vi "Target_long_compile.vi"() -> ()   [LabVIEW 2019]
uses:
  <vilib>/Platform/TimedLoop/XDataNode/timing_clust.ctl
  <vilib>/Platform/TimedLoop/XDataNode/nitl_modes.ctl
  <vilib>/Platform/TimedLoop/XDataNode/wakeup.ctl
  <vilib>/rvi/Emulation/niFpgaSctlEmulationGetInTimedLoop.vi
  <vilib>/rvi/Emulation/niFpgaEmulationReportErrorSimple.vi
  <vilib>/rvi/Emulation/niFpgaGetClockAttributes.vi
  <vilib>/rvi/Emulation/niFpgaCriticalErrorInLSC.vi
  <vilib>/rvi/DataTransferAndStorage/Container/Common/niFpgaContainerExecOnDevCompGetState.vi
  <vilib>/rvi/Emulation/niFpgaEmulationIsFPGAContextNoSignature.vi
  <vilib>/rvi/errors/niFpgaSetErrorForExecOnDevCompSimple.vi
  <vilib>/rvi/eio/common/nirviEmuReportErrorAndStop.vi
  <vilib>/rvi/DataTransferAndStorage/Container/Common/niFpgaContainerGetUniqueNameForEmu.vi
  <vilib>/rvi/FIFO/Fifo_Resource/nirvififoEmulationSetSize.vi
  <vilib>/rvi/FIFO/Fifo_Resource/nirviFifoEmulationQueueMgr.vi
  <instcachedir>/0/nirviFifoEmulationQueueMgr_E5CAEC123FF24DC58D834DCA3CDAA9B5.lvgen/nirviFifoEmulationQueueMgr_E5CAEC123FF24DC58D834DCA3CDAA9B5_006.vi
  <vilib>/rvi/FIFO/Fifo_Resource/nirvififoEmulationDetermineInputValidOut.vi
  <vilib>/rvi/FIFO/Fifo_Resource/nirvififoEmulationCreateLock.vi
  <vilib>/rvi/Emulation/niFpgaProcessEmulError.vi
  <vilib>/rvi/FIFO/Fifo_Resource/nirvififoEmulationObtainLock.vi
  <vilib>/rvi/FIFO/Fifo_Resource/nirvififoEmulationReleaseLock.vi
  <vilib>/rvi/occurrence/nirviWaitOnOccurrenceBase.vi
  <vilib>/rvi/errors/nirviReportUnexpectedCaseInternalError.vi
  <vilib>/rvi/errors/nirviReportUnexpectedCaseInternalError (U32).vi
  <vilib>/Utility/error.llb/Clear Errors.vi
  <vilib>/rvi/interface/RandomDataEmulation/niFpgaRandomDataHandleErrors.vi
  <vilib>/platform/TimedLoop/XDataNode/XDataNode.xnode
  <vilib>/rvi/DataTransferAndStorage/Container/XNode/niFpgaContainer.xnode
  <vilib>/rvi/FIFO/Fifo_Resource/niFpgaFifoEmulationRefIn.vi
  <vilib>/Platform/TimedLoop/XDataNode/XDNodeRunTimeDep.lvlib
panel:
  out "T5":u32 caption="Tick Count(mSec)"
  out "T4":u32 caption="Tick Count(mSec)"
  out "T3":u32 caption="Tick Count(mSec)"
  out "T2":u32 caption="Tick Count(mSec)"
  out "T1":u32 caption="Tick Count(mSec)"
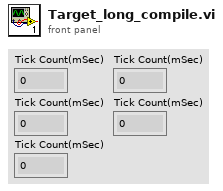
[diagram p1: front panel]
types:
  T1 = typedef "XDNodeRunTimeDep.lvlib/timing_clust.ctl" = cluster{"Expected End [f-1]":u64, "Actual End [f-1]":u64, "Finished Late? [f-1]":bool, "Expected End [i-1]":u64, "Actual End [i-1]":u64, "Finished Late? [i-1]":bool, "Expected Start [i]":u64, "Actual Start [i]":u64, "Expected Start [f]":u64, "Actual Start [f]":u64, "Source Name":string, "Structure Name":string, "Period":i64, "Deadline":i64, "Offset":i64, "Start":i64, "Priority":i32, "Timeout":i32, "Mode":T2, "Wakeup Reason":T3, "Error":errorcluster, "Source Type":string, "Secondary Source Type":string, "Global End Time":u64, "Global Start Time":u64, "Frame Duration":u64, "Iteration Duration":u64, "Assigned CPU":i32, "I/O Scan Engine Mode":u32}
  T2 = typedef "XDNodeRunTimeDep.lvlib/nitl_modes.ctl" = enum32{"No Change", "Process missed periods, maintain original phase", "Discard missed periods, maintain original phase", "Process missed periods, ignore original phase", "Discard missed periods, ignore original phase"}
  T3 = typedef "XDNodeRunTimeDep.lvlib/wakeup.ctl" = enum32{"Normal", "Aborted", "Asynchronous wakeup", "Timing source error", "Timed loop error", "Timeout"}
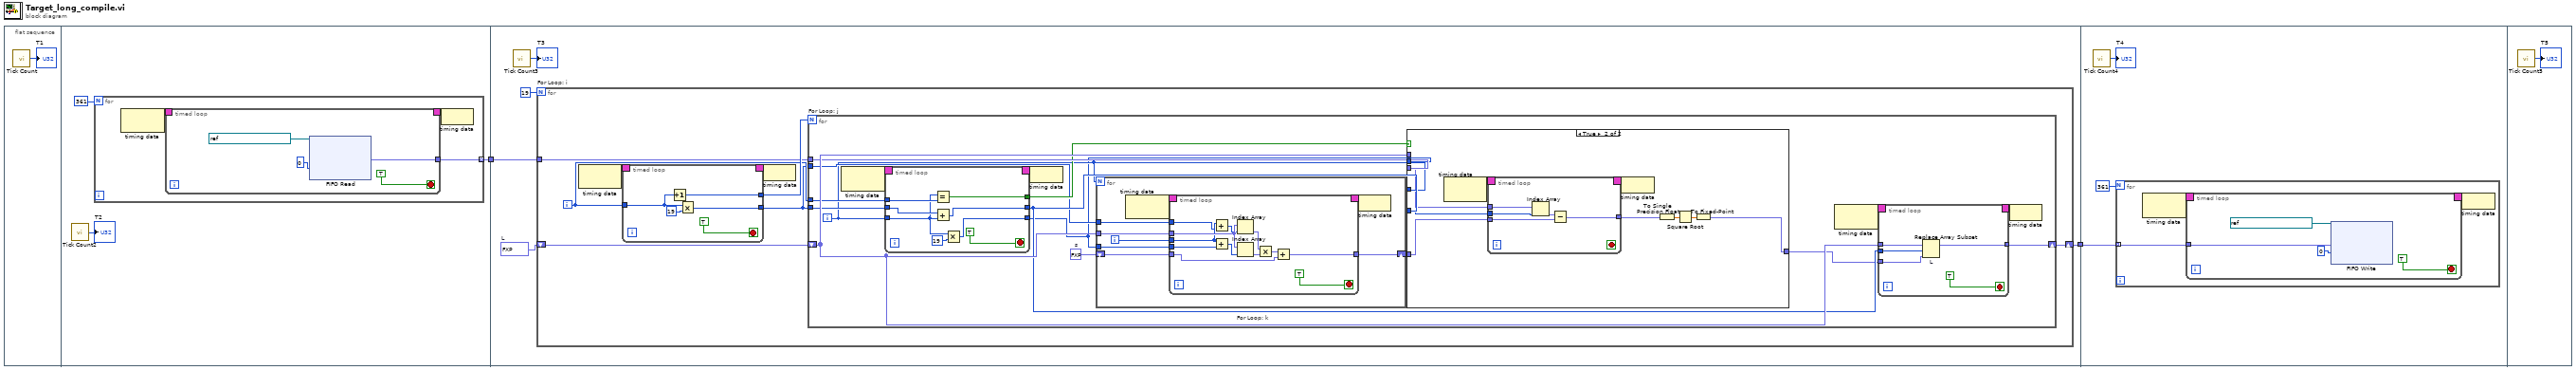
[diagram p0: block diagram]
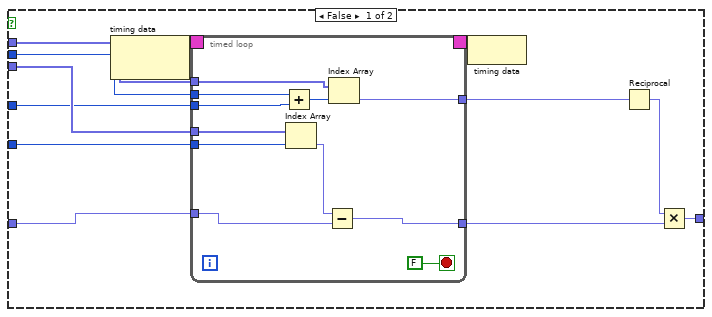
[diagram p2: hidden frame]
diagram:
  n1 = flat-sequence {
    tunnel: [w5] -> w2
    tunnel: w2 -> [w22]
    tunnel: [w21] -> w1
    tunnel: w1 -> [w148]
    frame #0 {
      n2 = call "Tick Count"() -> ("Tick Count(mSec)"=→"T1":u32)
    }
    frame #1 {
      n3 = call "Tick Count2"() -> ("Tick Count(mSec)"=→"T2":u32)
      n4 = for {
        N: 361 -> [_]
        tunnel: [w9] -> w5 mode=indexing
        n5 = node-c288() -> (w8:T1)  [unwired: 1 in]
        n6 = timed-loop {
          timing: w8 -> [_]
          timing-out: [_] -> w7
          tunnel: [w10] -> w9
          stop <- TRUE stop-if-true
          n7 = xnode ("FIFO Read")("Timeout"=0, "FIFO In"=refnum<k21> "FIFO-host-to-Cholesky") -> ("Element"=w10:fxp<+/-,32,0>)  [unwired: 2 out]
        }
        n8 = node-c288(w7) -> ()
      }
    }
    frame #2 {
      w20 = fxp<+,1,1>[] [0.0, 0.0, 0.0, 0.0, 0.0, 0.0, 0.0, 0.0, 0.0, 0.0, 0.0, 0.0, 0.0, 0.0, 0.0, 0.0, 0.0, 0.0, 0.0, 0.0, 0.0, 0.0, 0.0, 0.0, 0.0, 0.0, 0.0, 0.0, 0.0, 0.0, 0.0, 0.0, 0.0, 0.0, 0.0, 0.0, 0.0, 0.0, 0.0, 0.0, 0.0, 0.0, 0.0, 0.0, 0.0, 0.0, 0.0, 0.0, 0.0, 0.0, 0.0, 0.0, 0.0, 0.0, 0.0, 0.0, 0.0, 0.0, 0.0, 0.0, 0.0, 0.0, 0.0, 0.0, 0.0, 0.0, 0.0, 0.0, 0.0, 0.0, 0.0, 0.0, 0.0, 0.0, 0.0, 0.0, 0.0, 0.0, 0.0, 0.0, 0.0, 0.0, 0.0, 0.0, 0.0, 0.0, 0.0, 0.0, 0.0, 0.0, 0.0, 0.0, 0.0, 0.0, 0.0, 0.0, 0.0, 0.0, 0.0, 0.0, 0.0, 0.0, 0.0, 0.0, 0.0, 0.0, 0.0, 0.0, 0.0, 0.0, 0.0, 0.0, 0.0, 0.0, 0.0, 0.0, 0.0, 0.0, 0.0, 0.0, 0.0, 0.0, 0.0, 0.0, 0.0, 0.0, 0.0, 0.0, 0.0, 0.0, 0.0, 0.0, 0.0, 0.0, 0.0, 0.0, 0.0, 0.0, 0.0, 0.0, 0.0, 0.0, 0.0, 0.0, 0.0, 0.0, 0.0, 0.0, 0.0, 0.0, 0.0, 0.0, 0.0, 0.0, 0.0, 0.0, 0.0, 0.0, 0.0, 0.0, 0.0, 0.0, 0.0, 0.0, 0.0, 0.0, 0.0, 0.0, 0.0, 0.0, 0.0, 0.0, 0.0, 0.0, 0.0, 0.0, 0.0, 0.0, 0.0, 0.0, 0.0, 0.0, 0.0, 0.0, 0.0, 0.0, 0.0, 0.0, 0.0, 0.0, 0.0, 0.0, 0.0, 0.0, 0.0, 0.0, 0.0, 0.0, 0.0, 0.0, 0.0, 0.0, 0.0, 0.0, 0.0, 0.0, 0.0, 0.0, 0.0, 0.0, 0.0, 0.0, 0.0, 0.0, 0.0, 0.0, 0.0, 0.0, 0.0, 0.0, 0.0, 0.0, 0.0, 0.0, 0.0, 0.0, 0.0, 0.0, 0.0, 0.0, 0.0, 0.0, 0.0, 0.0, 0.0, 0.0, 0.0, 0.0, 0.0, 0.0, 0.0, 0.0, 0.0, 0.0, 0.0, 0.0, 0.0, 0.0, 0.0, 0.0, 0.0, 0.0, 0.0, 0.0, 0.0, 0.0, 0.0, 0.0, 0.0, 0.0, 0.0, 0.0, 0.0, 0.0, 0.0, 0.0, 0.0, 0.0, 0.0, 0.0, 0.0, 0.0, 0.0, 0.0, 0.0, 0.0, 0.0, 0.0, 0.0, 0.0, 0.0, 0.0, 0.0, 0.0, 0.0, 0.0, 0.0, 0.0, 0.0, 0.0, 0.0, 0.0, 0.0, 0.0, 0.0, 0.0, 0.0, 0.0, 0.0, 0.0, 0.0, 0.0, 0.0, 0.0, 0.0, 0.0, 0.0, 0.0, 0.0, 0.0, 0.0, 0.0, 0.0, 0.0, 0.0, 0.0, 0.0, 0.0, 0.0, 0.0, 0.0, 0.0, 0.0, 0.0, 0.0, 0.0, 0.0, 0.0, 0.0, 0.0, 0.0, 0.0, 0.0, 0.0, 0.0, 0.0, 0.0, 0.0, 0.0, 0.0, 0.0, 0.0, 0.0, 0.0, 0.0, 0.0, 0.0, 0.0, 0.0, 0.0, 0.0, 0.0, 0.0, 0.0, 0.0, 0.0, 0.0, 0.0, 0.0, 0.0, 0.0]  # L
      n9 = call "Tick Count3"() -> ("Tick Count(mSec)"=→"T3":u32)
      n10 = for "For Loop: i" {
        N: 19 -> [_]
        shift-right: [w28] -> w21
        shift-left: w20 -> [w30]
        tunnel: w22 -> [w27]
        i -> [w26]
        n11 = node-c288() -> (w24:T1)  [unwired: 1 in]
        n12 = timed-loop {
          timing: w24 -> [_]
          timing-out: [_] -> w23
          tunnel: [w35] -> w29
          tunnel: w26 -> [w33]
          tunnel: [w32] -> w25
          stop <- TRUE stop-if-true
          n13 = Increment(x=w33) -> (x+1=w35:i32)
          n14 = Multiply(x=w33, y=19) -> (x*y=w32:i32)
        }
        n15 = node-c288(w23) -> ()
        n16 = for "For Loop: j" {
          N: w29 -> [_]
          tunnel: w26 -> [w52]
          shift-right: [w54] -> w28
          shift-left: w30 -> [w53]
          tunnel: w27 -> [w51]
          tunnel: w25 -> [w46]
          tunnel: w25 -> [w45]
          i -> [w44]
          w56 = fxp<+,1,1> 0.0  # s
          n17 = node-c288() -> (w42:T1)  [unwired: 1 in]
          n18 = timed-loop {
            timing: w42 -> [_]
            timing-out: [_] -> w41
            tunnel: w52 -> [w64]
            tunnel: [w63] -> w50
            tunnel: w44 -> [w59]
            tunnel: [w58] -> w43
            tunnel: w46 -> [w61]
            tunnel: [w62] -> w49
            stop <- TRUE stop-if-true
            n19 = Equal?(x=w59, y=w64) -> (x = y?=w63:bool)
            n20 = Add(x=w61, y=w59) -> (x+y=w62:i32)
            n21 = Multiply(x=w59, y=19) -> (x*y=w58:i32)
          }
          n22 = node-c288(w41) -> ()
          n23 = for "For Loop: k" {
            N: w44 -> [_]
            tunnel: w53 -> [w130]
            shift-right: [w128] -> w55
            shift-left: w56 -> [w129]
            tunnel: w45 -> [w126]
            tunnel: w43 -> [w125]
            i -> [w127]
            n24 = node-c288() -> (w124:T1)  [unwired: 1 in]
            n25 = timed-loop {
              timing: w124 -> [_]
              timing-out: [_] -> w123
              tunnel: w130 -> [w141]
              tunnel: w127 -> [w134]
              tunnel: w126 -> [w133]
              tunnel: w125 -> [w132]
              tunnel: w129 -> [w138]
              tunnel: [w137] -> w128
              stop <- TRUE stop-if-true
              n26 = Add(x=w134, y=w133) -> (x+y=w136:i32)
              n27 = Add(x=w134, y=w132) -> (x+y=w135:i32)
              n28 = Index Array(array=w141, index=w136) -> (element=w142:fxp<+,1,1>)
              n29 = Index Array(array=w141, index=w135) -> (element=w140:fxp<+,1,1>)
              n30 = Multiply(x=w142, y=w140) -> (x*y=w139:fxp<+,1,1>)
              n31 = Add(x=w139, y=w138) -> (x+y=w137:fxp<+,1,1>)
            }
            n32 = node-c288(w123) -> ()
          }
          n33 = case shown="True" w50 {
            tunnel: w55 -> [w81 w113]
            tunnel: w53 -> [w89 _]
            tunnel: w51 -> [w86 w112]
            tunnel: w49 -> [w85 w111]
            tunnel: w44 -> [w84 _]
            tunnel: w43 -> [w83 _]
            tunnel: [w82 w110] -> w40
            frame False {
              n34 = node-c288() -> (w79:T1)  [unwired: 1 in]
              n35 = timed-loop {
                timing: w79 -> [_]
                timing-out: [_] -> w78
                tunnel: w89 -> [w100]
                tunnel: [w99] -> w88
                tunnel: w86 -> [w98]
                tunnel: w85 -> [w97]
                tunnel: w84 -> [w96]
                tunnel: w83 -> [w95]
                tunnel: w81 -> [w92]
                tunnel: [w91] -> w80
                stop <- FALSE stop-if-true
                n36 = Add(x=w95, y=w96) -> (x+y=w94:i32)
                n37 = Index Array(array=w98, index=w97) -> (element=w93:fxp<+/-,32,0>)
                n38 = Subtract(x=w93, y=w92) -> (x-y=w91:fxp<+/-,32,0>)
                n39 = Index Array(array=w100, index=w94) -> (element=w99:fxp<+,1,1>)
              }
              n40 = node-c288(w78) -> ()
              n41 = Reciprocal(x=w88) -> (1/x=w87:fxp<+,2,1>)
              n42 = Multiply(x=w87, y=w80) -> (x*y=w82:fxp<+/-,33,0>)
            }
            frame True {
              n43 = node-c288() -> (w106:T1)  [unwired: 1 in]
              n44 = timed-loop {
                timing: w106 -> [_]
                timing-out: [_] -> w105
                tunnel: w113 -> [w118]
                tunnel: w112 -> [w117]
                tunnel: w111 -> [w116]
                tunnel: [w114] -> w108
                stop <- _ stop-if-true
                n45 = Index Array(array=w117, index=w116) -> (element=w115:fxp<+/-,32,0>)
                n46 = Subtract(x=w115, y=w118) -> (x-y=w114:fxp<+/-,32,0>)
              }
              n47 = node-c288(w105) -> ()
              n48 = To Single Precision Float(number=w108) -> (single precision float=w107:sgl)
              n49 = Square Root(x=w107) -> (sqrt(x)=w109:sgl)
              n50 = To Fixed-Point(number=w109) -> (fixed-point=w110:fxp<+/-,32,16>)  [unwired: 1 in]
            }
          }
          n51 = node-c288() -> (w48:T1)  [unwired: 1 in]
          n52 = timed-loop {
            timing: w48 -> [_]
            timing-out: [_] -> w47
            tunnel: w49 -> [w71]
            tunnel: w40 -> [w69]
            tunnel: w53 -> [w72]
            tunnel: [w73] -> w54
            stop <- TRUE stop-if-true
            n53 = Replace Array Subset "L"(array=w72, new element=w69, index=w71) -> (w73:fxp<+,1,1>[])
          }
          n54 = node-c288(w47) -> ()
        }
      }
    }
    frame #3 {
      n55 = call "Tick Count4"() -> ("Tick Count(mSec)"=→"T4":u32)
      n56 = for {
        N: 361 -> [_]
        tunnel: w148 -> [w152] mode=indexing
        n57 = node-c288() -> (w151:T1)  [unwired: 1 in]
        n58 = timed-loop {
          tunnel: w152 -> [w153]
          timing: w151 -> [_]
          timing-out: [_] -> w150
          stop <- TRUE stop-if-true
          n59 = xnode ("FIFO Write")("Element"=w153, "Timeout"=0, "FIFO In"=refnum<k21> "FIFO-Cholesky-to-host") -> ()  [unwired: 2 out]
        }
        n60 = node-c288(w150) -> ()
      }
    }
    frame #4 {
      n61 = call "Tick Count5"() -> ("Tick Count(mSec)"=→"T5":u32)
    }
  }
